vi "WPI_AccelerometerGetAcceleration.vi"(8 "error in":errorcluster, 11 "AccelerometerDevRef":T2={"DevStatus"={"status"=FALSE, "code"=0, "source"=""}, "Scaling"={"Gain (VoltsPerG)"=0.0, "Center Voltage"=0.0}, "Analog Channels"={"X-Axis"=enum."Invalid", "Y-Axis"=enum."Invalid", "Z-Axis"=enum."Invalid"}, "I2C Bus"=enum."Invalid", "SPI Bus"=enum."Invalid", "Accel Range"=0, "ADXL Axes"={"X-Axis"=FALSE, "Y-Axis"=FALSE, "Z-Axis"=FALSE}, "Handle"=0, "Device Address"=0, "Accel Type"=enum."Analog"} {"Device Address" format="%.0x"; "Accel Range" items=["+/- 2 g", "+/- 4 g", "+/- 8 g", "+/- 16 g"]}) -> (0 "error out":errorcluster, 2 "Accelerations":T1, 3 "AccelerometerDevRef":T2={"DevStatus"={"status"=FALSE, "code"=0, "source"=""}, "Scaling"={"Gain (VoltsPerG)"=0.0, "Center Voltage"=0.0}, "Analog Channels"={"X-Axis"=enum."Invalid", "Y-Axis"=enum."Invalid", "Z-Axis"=enum."Invalid"}, "I2C Bus"=enum."Invalid", "SPI Bus"=enum."Invalid", "Accel Range"=0, "ADXL Axes"={"X-Axis"=FALSE, "Y-Axis"=FALSE, "Z-Axis"=FALSE}, "Handle"=0, "Device Address"=0, "Accel Type"=enum."Analog"} {"Device Address" format="%.0x"; "Accel Range" items=["+/- 2 g", "+/- 4 g", "+/- 8 g", "+/- 16 g"]})   [LabVIEW 2017]
doc: "Returns the current accelerations of the sensor that you specify.\n\nThis software is licensed. Open the labview\\readme\\WPI Robotics Library Open Source License.txt file for more information."
uses:
  <vilib>/Rock Robotics/WPI/Accelerometer/WPI_AccelerometerDevRef.ctl
  <vilib>/Rock Robotics/WPI/Accelerometer/WPI_AccelerometerScaling.ctl
  <vilib>/Rock Robotics/WPI/Accelerometer/WPI_AccelerometerAnalogChannels.ctl
  <vilib>/Rock Robotics/SystemInterfaces/AI/FPGA_AIChannel.ctl
  <vilib>/Rock Robotics/SystemInterfaces/i2clib/i2c_bus.ctl
  <vilib>/Rock Robotics/SystemInterfaces/spilib/spi_bus.ctl
  <vilib>/Rock Robotics/WPI/Accelerometer/ADXL345 Range.ctl
  <vilib>/Rock Robotics/WPI/Accelerometer/WPI_AccelerometerADXL345 Axes.ctl
panel:
  # "ADXL"
  # "Analog"
  # "ADXL"
  # "Analog"
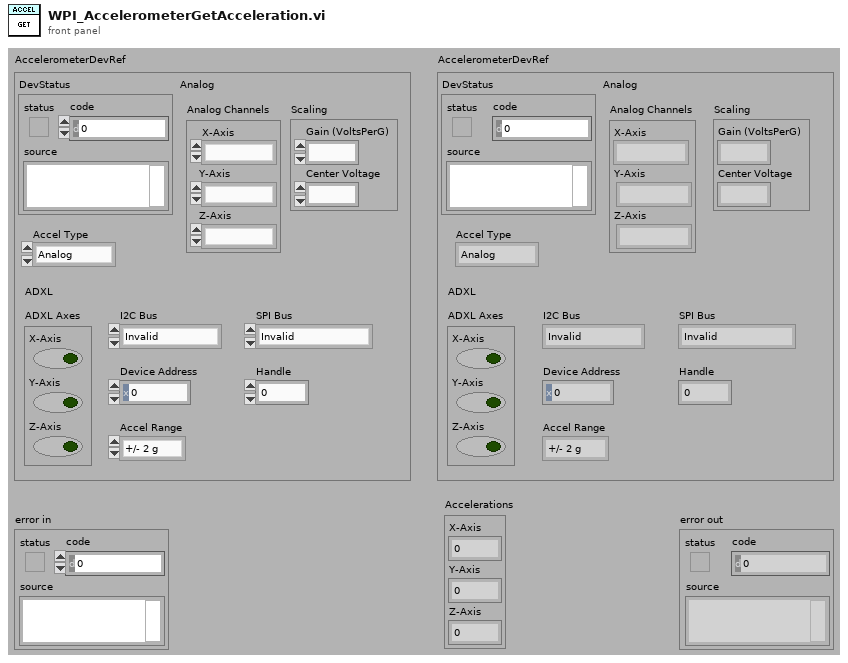
[diagram p1: front panel]
types:
  T1 = cluster{"X-Axis":dbl, "Y-Axis":dbl, "Z-Axis":dbl}
  T2 = typedef "WPI_AccelerometerDevRef.ctl" = cluster{"DevStatus":errorcluster, "Scaling":T3, "Analog Channels":T4, "I2C Bus":T6, "SPI Bus":T7, "Accel Range":T8, "ADXL Axes":T9, "Handle":i32, "Device Address":u8, "Accel Type":enum16{"Analog", "ADXL345 I2C", "ADXL345 SPI", "Internal", "ADXL362 SPI"}}
  T3 = typedef "WPI_AccelerometerScaling.ctl" = cluster{"Gain (VoltsPerG)":dbl, "Center Voltage":dbl}
  T4 = typedef "WPI_AccelerometerAnalogChannels.ctl" = cluster{"X-Axis":T5, "Y-Axis":T5, "Z-Axis":T5}
  T5 = typedef "FPGA_AIChannel.ctl" = enum8{"AI 0", "AI 1", "AI 2", "AI 3", "AI MXP 0", "AI MXP 1", "AI MXP 2", "AI MXP 3", "Invalid"}
  T6 = typedef "i2c_bus.ctl" = enum16{"I2C On-Board", "I2C MXP", "Invalid"}
  T7 = typedef "spi_bus.ctl" = enum16{"SPI On-Board, CS0", "SPI On-Board, CS1", "SPI On-Board, CS2", "SPI On-Board, CS3", "SPI MXP", "Invalid"}
  T8 = typedef "ADXL345 Range.ctl" = u8
  T9 = typedef "WPI_AccelerometerADXL345 Axes.ctl" = cluster{"X-Axis":bool, "Y-Axis":bool, "Z-Axis":bool}
  T10 = enum16{"Analog", "ADXL345 I2C", "ADXL345 SPI", "Internal", "ADXL362 SPI"}
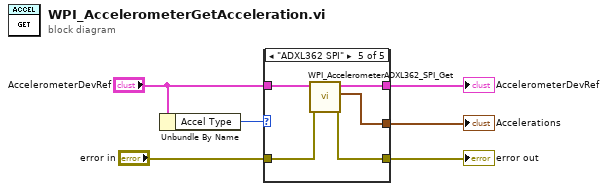
[diagram p0: block diagram]
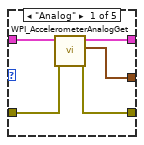
[diagram p2: hidden frame]
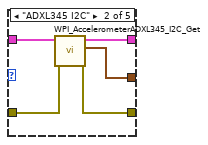
[diagram p3: hidden frame]
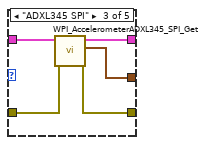
[diagram p4: hidden frame]
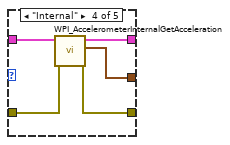
[diagram p5: hidden frame]
diagram:
  n1 = Unbundle By Name("AccelerometerDevRef") -> ("Accel Type"=w5:T10)
  n2 = case shown="\"ADXL362 SPI\"" w5 {
    tunnel: "AccelerometerDevRef" -> [w11 w16 w21 w26 w31]
    tunnel: [w10 w15 w20 w25 w30] -> w4
    tunnel: "error in" -> [w9 w14 w19 w24 w29]
    tunnel: [w8 w12 w17 w22 w27] -> w2
    tunnel: [w7 w13 w18 w23 w28] -> w1
    frame "Analog" {
      n3 = call <vilib>:"WPI_AccelerometerAnalogGet.vi"("error in"=w9, "AccelerometerDevRef"=w11) -> ("error out"=w7:errorcluster, "Accelerations"=w8:T1, "AccelerometerDevRef"=w10:T2)  [unwired: 7 in]
    }
    frame "ADXL345 I2C" {
      n4 = call <vilib>:"WPI_AccelerometerADXL345_I2C_Get.vi"("error in"=w14, "AccelerometerDevRef"=w16) -> ("error out"=w13:errorcluster, "Accelerations"=w12:T1, "AccelerometerDevRef"=w15:T2)  [unwired: 7 in]
    }
    frame "ADXL345 SPI" {
      n5 = call <vilib>:"WPI_AccelerometerADXL345_SPI_Get.vi"("error in"=w19, "AccelerometerDevRef"=w21) -> ("error out"=w18:errorcluster, "Accelerations"=w17:T1, "AccelerometerDevRef"=w20:T2)  [unwired: 7 in]
    }
    frame "Internal" {
      n6 = call <vilib>:"WPI_AccelerometerInternalGetAcceleration.vi"("error in"=w24, "AccelerometerDevRef"=w26) -> ("error out"=w23:errorcluster, "Accelerations"=w22:T1, "AccelerometerDevRef"=w25:T2)  [unwired: 7 in]
    }
    frame "ADXL362 SPI" {
      n7 = call <vilib>:"WPI_AccelerometerADXL362_SPI_Get.vi"("error in"=w29, "AccelerometerDevRef"=w31) -> ("error out"=w28:errorcluster, "Accelerations"=w27:T1, "AccelerometerDevRef"=w30:T2)  [unwired: 7 in]
    }
  }
  "AccelerometerDevRef" <- w4
  "error out" <- w1
  "Accelerations" <- w2
